vi "Write Bottom Segments.vi"(8 "error in (no error)":errorcluster, 10 "Bottom Segments":dbl, 11 "Funnel Settings in":refnum<class "Funnel Settings.lvclass">) -> (0 "error out":errorcluster, 3 "Funnel Settings out":refnum<class "Funnel Settings.lvclass">)   [LabVIEW 2019, in "Funnel Settings.lvclass"]
uses:
  Funnel Settings.lvclass
  Funnel Settings.lvclass/Funnel Settings.ctl
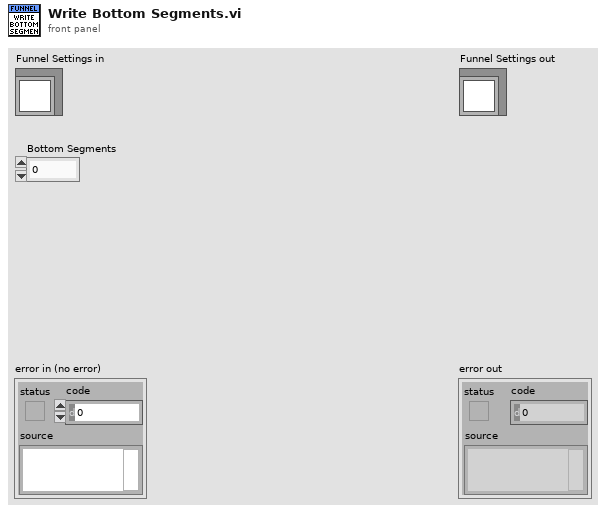
[diagram p1: front panel]
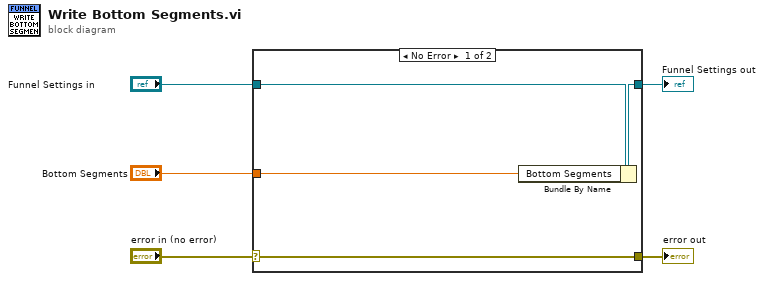
[diagram p0: block diagram]
diagram:
  n1 = case shown="No Error" "error in (no error)" {
    selector: "error in (no error)" -> [w9 w10]
    tunnel: [w9 w10] -> w4
    tunnel: [w7 w11] -> w2
    tunnel: "Funnel Settings in" -> [w8 w11]
    tunnel: "Bottom Segments" -> [w6 _]
    frame No Error {
      n2 = Bundle By Name(cluster=w8, "Bottom Segments"=w6) -> (w7:refnum<class "Funnel Settings.lvclass">)
    }
    frame Error {
    }
  }
  "error out" <- w4
  "Funnel Settings out" <- w2
